vi "variant2Attributes.vi"(0 "HGF_DIMBaseType":refnum<class "HGF_DIMDataConverter.lvclass">, 2 "rawData":variant, 3 "typeDescriptor":string, 5 "error in (no error)":errorcluster) -> (14 "HGF_DIMBaseType":refnum<class "HGF_DIMDataConverter.lvclass">, 15 "no link":bool, 16 "Parameter":variant, 17 "typeDescriptor":string, 19 "error out":errorcluster)   [LabVIEW 2012, in "HGF_DIM.lvlib" / "HGF_DIMDataConverter.lvclass"]
doc: "Convert raw data value of variant to variant attributes Pn, n=0,1,2,..."
uses:
  HGF_DIMDataConverter.lvclass
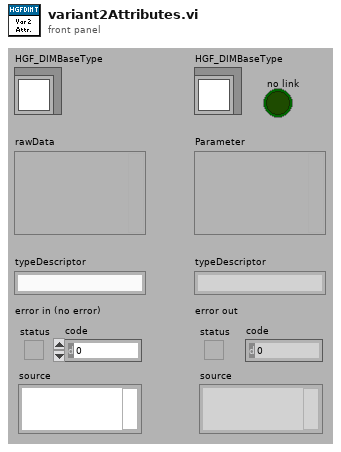
[diagram p1: front panel]
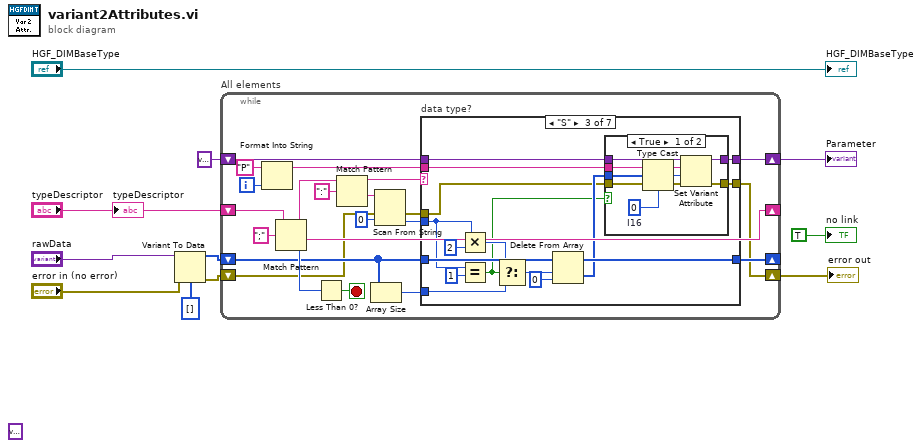
[diagram p0: block diagram]
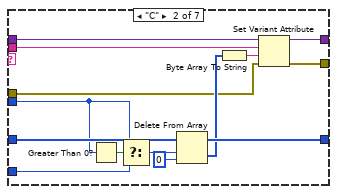
[diagram p3: hidden frame]
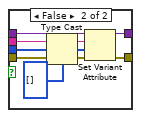
[diagram p4: hidden frame]
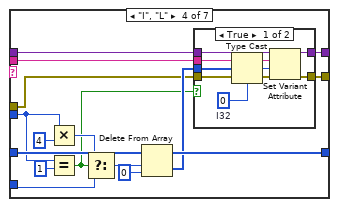
[diagram p5: hidden frame]
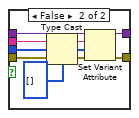
[diagram p6: hidden frame]
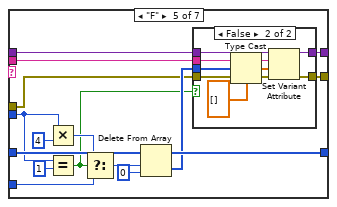
[diagram p7: hidden frame]
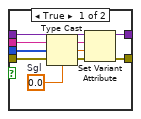
[diagram p8: hidden frame]
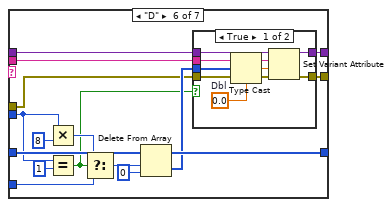
[diagram p9: hidden frame]
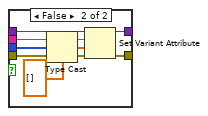
[diagram p10: hidden frame]
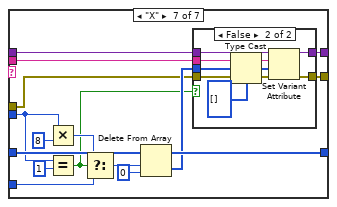
[diagram p11: hidden frame]
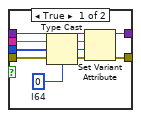
[diagram p12: hidden frame]
diagram:
  (unwired) variant ("rawData")
  (unwired) variant ("rawData")
  n1 = Variant To Data(error in="error in (no error)", type=i8[] [], Variant="rawData") -> (data=w8:i8[], error out=w3:errorcluster)
  n2 = while "All elements" {
    shift-right: [w31] -> _
    shift-left: "typeDescriptor" -> [w33]
    shift-right: [w25] -> w6
    shift-left: variant ("rawData") -> [w26]
    shift-right: [w21] -> _
    shift-left: w8 -> [w16]
    shift-right: [w12] -> w2
    shift-left: w3 -> [w14]
    i -> [w23]
    stop <- w30 stop-if-true
    n3 = Format Into String(initial string="P", w23) -> (resulting string=w22:string)  [unwired: 2 in, 1 out]
    n4 = Match Pattern(string=w33, regular expression=";") -> (before substring=w28:string, after substring=w31:string, offset past match=w29:i32)  [unwired: 2 out]
    n5 = Less Than 0?(x=w29) -> (x < 0?=w30:bool)
    n6 = Match Pattern(string=w28, regular expression=":") -> (before substring=w20:string, after substring=w18:string)  [unwired: 3 out]
    n7 = Array Size(array=w16) -> (size(s)=w15:i32)
    n8 = Scan From String(input string=w18, error in=w14, default 1=0 ("default value 1")) -> (error out=w13:errorcluster, output 1=w17:i32)  [unwired: 2 in, 2 out]
    n9 = case "data type?" shown="\"S\"" w20 {
      tunnel: w26 -> [w36 w50 w66 w98 w130 w162 w194]
      tunnel: [w36 w49 w65 w97 w129 w161 w193] -> w25
      tunnel: w22 -> [_ w48 w64 w96 w128 w160 w192]
      tunnel: w16 -> [w35 w43 w60 w92 w124 w156 w188]
      tunnel: [w35 w44 w61 w93 w125 w157 w189] -> w21
      tunnel: w17 -> [_ w40 w53 w86 w118 w150 w182]
      tunnel: w15 -> [_ w39 w54 w85 w117 w149 w181]
      tunnel: w13 -> [w34 w37 w52 w84 w116 w148 w180]
      tunnel: [w34 w38 w51 w83 w115 w147 w179] -> w12
      frame Default {
      }
      frame "C" {
        n10 = Greater Than 0?(x=w40) -> (x > 0?=w42:bool)
        n11 = Select(t=w40, s=w42, f=w39) -> (s? t:f=w45:i32)
        n12 = Delete From Array(array=w43, length=w45, index=0) -> (deleted portion=w41:i8[], array with subset deleted=w44:i8[])
        n13 = Byte Array To String(unsigned byte array=w41) -> (string=w47:string)
        n14 = Set Variant Attribute(Variant=w50, name=w48, value=w47, error in=w37) -> (Variant out=w49:variant, error out=w38:errorcluster)  [unwired: 1 out]
      }
      frame "S" {
        n15 = Multiply(x=w53, y=2) -> (x*y=w58:i32)
        n16 = Equal?(x=w53, y=1) -> (x = y?=w56:bool)
        n17 = Select(t=w58, s=w56, f=w54) -> (s? t:f=w62:i32)
        n18 = Delete From Array(array=w60, length=w62, index=0) -> (deleted portion=w57:i8[], array with subset deleted=w61:i8[])
        n19 = case shown="True" w56 {
          tunnel: w66 -> [w74 w82]
          tunnel: [w73 w81] -> w65
          tunnel: w64 -> [w72 w80]
          tunnel: w57 -> [w70 w79]
          tunnel: w52 -> [w68 w76]
          tunnel: [w67 w75] -> w51
          frame True {
            w71 = i16 0  # I16
            n20 = Type Cast(type=w71, x=w70) -> (*(type *) &x=w69:i16)
            n21 = Set Variant Attribute(Variant=w74, name=w72, value=w69, error in=w68) -> (Variant out=w73:variant, error out=w67:errorcluster)  [unwired: 1 out]
          }
          frame False {
            n22 = Type Cast(type=i16[] [], x=w79) -> (*(type *) &x=w78:i16[])
            n23 = Set Variant Attribute(Variant=w82, name=w80, value=w78, error in=w76) -> (Variant out=w81:variant, error out=w75:errorcluster)  [unwired: 1 out]
          }
        }
      }
      frame "I", "L" {
        n24 = Multiply(x=w86, y=4) -> (x*y=w90:i32)
        n25 = Equal?(x=w86, y=1) -> (x = y?=w88:bool)
        n26 = Select(t=w90, s=w88, f=w85) -> (s? t:f=w94:i32)
        n27 = Delete From Array(array=w92, length=w94, index=0) -> (deleted portion=w89:i8[], array with subset deleted=w93:i8[])
        n28 = case shown="True" w88 {
          tunnel: w98 -> [w106 w114]
          tunnel: [w105 w113] -> w97
          tunnel: w96 -> [w104 w112]
          tunnel: w89 -> [w102 w111]
          tunnel: w84 -> [w99 w108]
          tunnel: [w100 w107] -> w83
          frame True {
            w103 = 0  # I32
            n29 = Type Cast(type=w103, x=w102) -> (*(type *) &x=w101:i32)
            n30 = Set Variant Attribute(Variant=w106, name=w104, value=w101, error in=w99) -> (Variant out=w105:variant, error out=w100:errorcluster)  [unwired: 1 out]
          }
          frame False {
            n31 = Type Cast(type=i32[] [], x=w111) -> (*(type *) &x=w110:i32[])
            n32 = Set Variant Attribute(Variant=w114, name=w112, value=w110, error in=w108) -> (Variant out=w113:variant, error out=w107:errorcluster)  [unwired: 1 out]
          }
        }
      }
      frame "F" {
        n33 = Multiply(x=w118, y=4) -> (x*y=w122:i32)
        n34 = Equal?(x=w118, y=1) -> (x = y?=w120:bool)
        n35 = Select(t=w122, s=w120, f=w117) -> (s? t:f=w126:i32)
        n36 = Delete From Array(array=w124, length=w126, index=0) -> (deleted portion=w121:i8[], array with subset deleted=w125:i8[])
        n37 = case shown="False" w120 {
          tunnel: w130 -> [w138 w146]
          tunnel: [w137 w145] -> w129
          tunnel: w128 -> [w136 w144]
          tunnel: w121 -> [w134 w143]
          tunnel: w116 -> [w132 w140]
          tunnel: [w131 w139] -> w115
          frame True {
            w135 = sgl 0.0  # Sgl
            n38 = Type Cast(type=w135, x=w134) -> (*(type *) &x=w133:sgl)
            n39 = Set Variant Attribute(Variant=w138, name=w136, value=w133, error in=w132) -> (Variant out=w137:variant, error out=w131:errorcluster)  [unwired: 1 out]
          }
          frame False {
            n40 = Type Cast(type=sgl[] [], x=w143) -> (*(type *) &x=w142:sgl[])
            n41 = Set Variant Attribute(Variant=w146, name=w144, value=w142, error in=w140) -> (Variant out=w145:variant, error out=w139:errorcluster)  [unwired: 1 out]
          }
        }
      }
      frame "D" {
        n42 = Multiply(x=w150, y=8) -> (x*y=w154:i32)
        n43 = Equal?(x=w150, y=1) -> (x = y?=w152:bool)
        n44 = Select(t=w154, s=w152, f=w149) -> (s? t:f=w158:i32)
        n45 = Delete From Array(array=w156, length=w158, index=0) -> (deleted portion=w153:i8[], array with subset deleted=w157:i8[])
        n46 = case shown="True" w152 {
          tunnel: w162 -> [w170 w178]
          tunnel: [w169 w177] -> w161
          tunnel: w160 -> [w168 w176]
          tunnel: w153 -> [w166 w175]
          tunnel: w148 -> [w164 w172]
          tunnel: [w163 w171] -> w147
          frame True {
            w167 = 0.0  # Dbl
            n47 = Type Cast(type=w167, x=w166) -> (*(type *) &x=w165:dbl)
            n48 = Set Variant Attribute(Variant=w170, name=w168, value=w165, error in=w164) -> (Variant out=w169:variant, error out=w163:errorcluster)  [unwired: 1 out]
          }
          frame False {
            n49 = Type Cast(type=dbl[] [], x=w175) -> (*(type *) &x=w174:dbl[])
            n50 = Set Variant Attribute(Variant=w178, name=w176, value=w174, error in=w172) -> (Variant out=w177:variant, error out=w171:errorcluster)  [unwired: 1 out]
          }
        }
      }
      frame "X" {
        n51 = Multiply(x=w182, y=8) -> (x*y=w186:i32)
        n52 = Equal?(x=w182, y=1) -> (x = y?=w184:bool)
        n53 = Select(t=w186, s=w184, f=w181) -> (s? t:f=w190:i32)
        n54 = Delete From Array(array=w188, length=w190, index=0) -> (deleted portion=w185:i8[], array with subset deleted=w189:i8[])
        n55 = case shown="False" w184 {
          tunnel: w194 -> [w202 w210]
          tunnel: [w201 w209] -> w193
          tunnel: w192 -> [w200 w208]
          tunnel: w185 -> [w198 w207]
          tunnel: w180 -> [w196 w204]
          tunnel: [w195 w203] -> w179
          frame True {
            w199 = i64 0  # I64
            n56 = Type Cast(type=w199, x=w198) -> (*(type *) &x=w197:i64)
            n57 = Set Variant Attribute(Variant=w202, name=w200, value=w197, error in=w196) -> (Variant out=w201:variant, error out=w195:errorcluster)  [unwired: 1 out]
          }
          frame False {
            n58 = Type Cast(type=i64[] [], x=w207) -> (*(type *) &x=w206:i64[])
            n59 = Set Variant Attribute(Variant=w210, name=w208, value=w206, error in=w204) -> (Variant out=w209:variant, error out=w203:errorcluster)  [unwired: 1 out]
          }
        }
      }
    }
  }
  "error out" <- w2
  "Parameter" <- w6
  "HGF_DIMBaseType" <- "HGF_DIMBaseType"
  "typeDescriptor" <- "typeDescriptor"
  "no link" <- TRUE ("no link")
